vi "Create_Error_log_folders.vi"(3 "Per Day Log File?":bool, 4 "Log Folder":string, 5 "Log Filename":string) -> (0 "exists?":bool, 1 "Server copy Location":path, 2 "Local Log File":path)   [LabVIEW 2017]
uses:
  Globals/Constants_global.vi
  Globals/Preference_global.vi
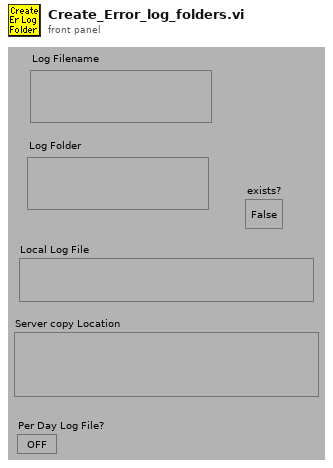
[diagram p1: front panel]
types:
  T1 = cluster{"second":i32, "minute":i32, "hour":i32, "day of month":i32, "month":i32, "year":i32, "day of week":i32, "day of year":i32, "is DST":i32}
  T2 = typedef "EnFlo_Data_Folder_Setup.ctl" = string
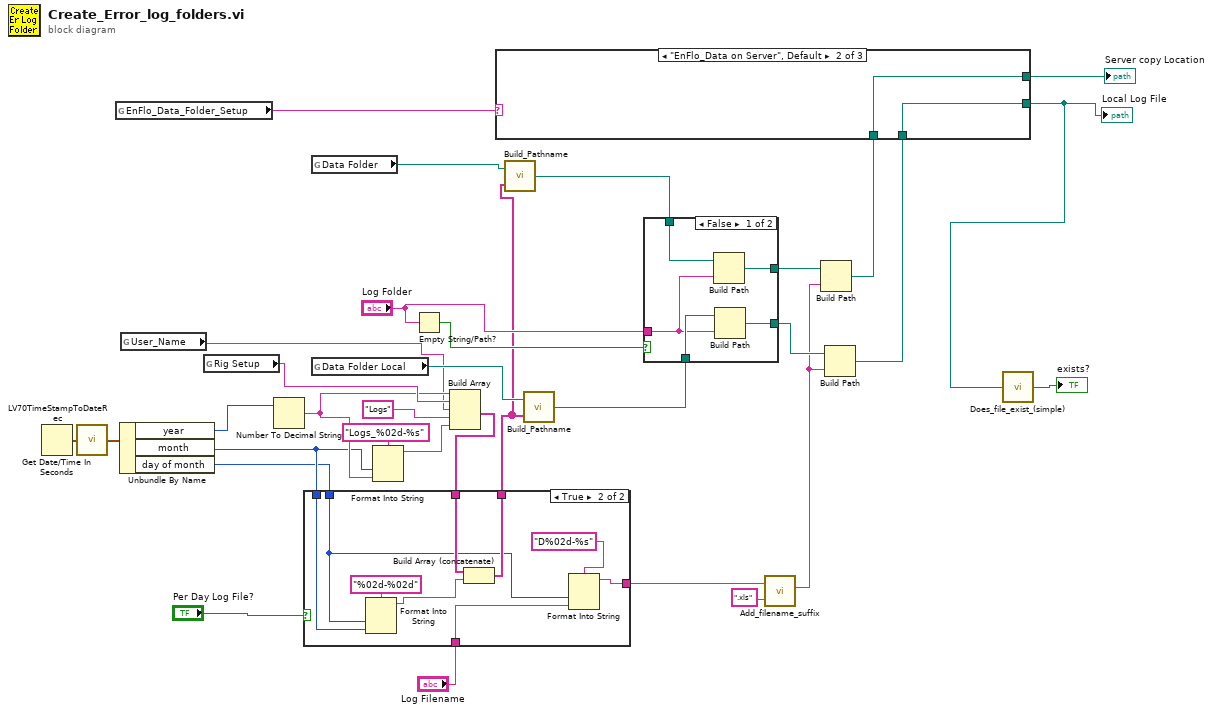
[diagram p0: block diagram]
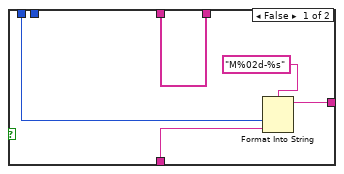
[diagram p4: hidden frame]
diagram:
  n1 = Get Date/Time In Seconds() -> (seconds since 1Jan1904=w11:timestamp)
  n2 = call <vilib>:"LV70TimeStampToDateRec.vi"("time stamp"=w11) -> ("date time rec"=w31:T1)
  n3 = global read "Preference_global.vi" "EnFlo_Data_Folder_Setup"() -> (w9:T2)
  n4 = Unbundle By Name(w31) -> ("year"=w30:i32, "month"=w4:i32, "day of month"=w3:i32)
  n5 = global read "Preference_global.vi" "User_Name"() -> (w10:string)
  n6 = global read "Preference_global.vi" "Rig Setup"() -> (w24:string)
  n7 = Number To Decimal String(number=w30) -> (decimal integer string=w22:string)  [unwired: 1 out]
  n8 = global read "Constants_global.vi" "Data Folder"() -> (w18:path)
  n9 = global read "Constants_global.vi" "Data Folder Local"() -> (w29:path)
  n10 = Format Into String(format string="Logs_%02d-%s", w4, w22) -> (resulting string=w20:string)  [unwired: 2 in, 1 out]
  n11 = Empty String/Path?(string/path="Log Folder") -> (empty?=w25:bool)
  n12 = Build Array(w22, w24, w10, "Logs", w20) -> (w13:string[])
  n13 = case shown="True" "Per Day Log File?" {
    tunnel: w3 -> [_ w38]
    tunnel: w13 -> [w37 w44]
    tunnel: [w37 w43] -> w12
    tunnel: w4 -> [w33 w42]
    tunnel: "Log Filename" -> [w35 w40]
    tunnel: [w34 w39] -> w1
    frame False {
      n14 = Format Into String(format string="M%02d-%s", w33, w35) -> (resulting string=w34:string)  [unwired: 2 in, 1 out]
    }
    frame True {
      n15 = Format Into String(format string="%02d-%02d", w38, w42) -> (resulting string=w45:string)  [unwired: 2 in, 1 out]
      n16 = Build Array (concatenate)(w44, w45) -> (w43:string[])
      n17 = Format Into String(format string="D%02d-%s", w38, w40) -> (resulting string=w39:string)  [unwired: 2 in, 1 out]
    }
  }
  n18 = call "Build_Pathname.vi"("PathElements"=w12, "PathnameIn"=w18) -> ("AppendedPath"=w17:path)
  n19 = call "Build_Pathname.vi"("PathElements"=w12, "PathnameIn"=w29) -> ("AppendedPath"=w27:path)
  n20 = case shown="False" w25 {
    tunnel: w27 -> [w51 w53]
    tunnel: [w50 w53] -> w32
    tunnel: "Log Folder" -> [w48 _]
    tunnel: w17 -> [w49 w52]
    tunnel: [w47 w52] -> w16
    frame False {
      n21 = Build Path(base path=w49, name or relative path=w48) -> (appended path=w47:path)
      n22 = Build Path(base path=w51, name or relative path=w48) -> (appended path=w50:path)
    }
    frame True {
    }
  }
  n23 = call "Add_filename_suffix.vi"("Filename"=w1, "Suffix to add"=".xls") -> ("Filename out"=w15:string)  [unwired: 3 out]
  n24 = Build Path(base path=w16, name or relative path=w15) -> (appended path=w7:path)
  n25 = Build Path(base path=w32, name or relative path=w15) -> (appended path=w6:path)
  n26 = case shown="\"EnFlo_Data on Server\", Default" w9 {
    tunnel: [w54 w56 w57] -> w8
    tunnel: w7 -> [w54 w56 w57]
    tunnel: [w54 w55 w57] -> w5
    tunnel: w6 -> [_ w55 _]
    frame "EnFlo_Data on C drive - do not backup" {
    }
    frame "EnFlo_Data on Server", Default {
    }
    frame "EnFlo_Data on C drive - backup to server" {
    }
  }
  "Local Log File" <- w5
  "Server copy Location" <- w8
  n27 = call "Does_file_exist_(simple).vi"("Pathname"=w5) -> ("exists?"=→"exists?":bool)
